vi "Write Tags.vi"(8 "error in (no error)":errorcluster, 11 "State in":T1={"State"=enum."Idle", "Start Time"=timestamp(0 s since 1904-01-01), "Configuration"={"Cycle Period"=0.0, "Mettler"={"VISA resource name"="", "Simulated?"=FALSE}, "Scale Type"=""}, "Current Time"=timestamp(0 s since 1904-01-01), "First Iteration"=FALSE, "Data"={"Scale Read(g)"=0.0}, "Process Name"="", "Log Started"=FALSE}) -> (0 "error out":errorcluster, 3 "State out":T1={"State"=enum."Idle", "Start Time"=timestamp(0 s since 1904-01-01), "Configuration"={"Cycle Period"=0.0, "Mettler"={"VISA resource name"="", "Simulated?"=FALSE}, "Scale Type"=""}, "Current Time"=timestamp(0 s since 1904-01-01), "First Iteration"=FALSE, "Data"={"Scale Read(g)"=0.0}, "Process Name"="", "Log Started"=FALSE})   [LabVIEW 2018, in "Scale Module.lvlib" / "Scale Module Engine.lvlib"]
uses:
  Scale Module Engine.lvlib
  State Cluster.ctl
  State Enum.ctl
  Feed Module/Controls/Scale Module Settings Cluster.ctl
  Mettler Toledo/Controls/Settings Cluster.ctl
  Tag VIs/Tag FGV Operation Enum.ctl
  Shared Variables/Dynamic Shared Variables.lvlib
  Scale Module.lvlib
  Mettler Toledo/Mettler Toledo.lvlib
panel:
  # "Scale Settings"
  # "Scale Settings"
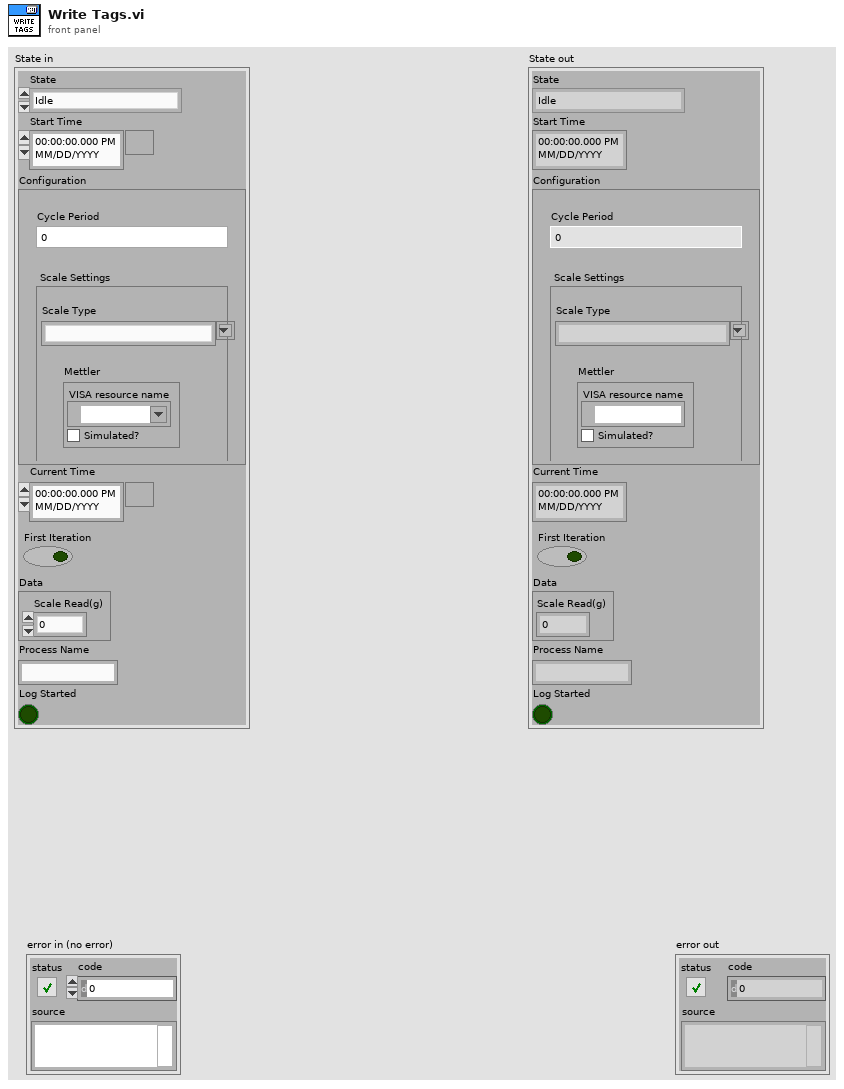
[diagram p1: front panel]
types:
  T1 = typedef "Scale Module.lvlib/Scale Module Engine.lvlib/State Cluster.ctl" = cluster{"State":T2, "Start Time":timestamp, "Configuration":T3, "Current Time":timestamp, "First Iteration":bool, "Data":cluster{"Scale Read(g)":dbl}, "Process Name":string, "Log Started":bool}
  T2 = typedef "Scale Module.lvlib/Scale Module Engine.lvlib/State Enum.ctl" = enum16{"Measuring", "Idle"}
  T3 = typedef "Scale Module.lvlib/Scale Module Settings Cluster.ctl" = cluster{"Cycle Period":dbl, "Mettler":T4, "Scale Type":string}
  T4 = typedef "Mettler Toledo.lvlib/Settings Cluster.ctl" = cluster{"VISA resource name":refnum<visa-resource-name>, "Simulated?":bool}
  T5 = typedef "Tag FGV Operation Enum.ctl" = enum16{"Init", "Set Notification Queue", "Create Tag", "Commit", "Write Tag (Numeric)", "Write Tag (Boolean)", "Read All Tags", "Read One Tag", "Delete Tag Category", "Set Alarm Parameters (Numeric)", "Set Alarm Parameters (Boolean)", "Enable All Alarms", "Disable All Alarms", "Delete All Tags", "Read Alarms", "Ack Alarm", "Read Alarm Parameters (Numeric)", "Read Alarm Parameters (Boolean)"}
  T6 = cluster{"Scale Tag":string, "Output Device Tag":string}
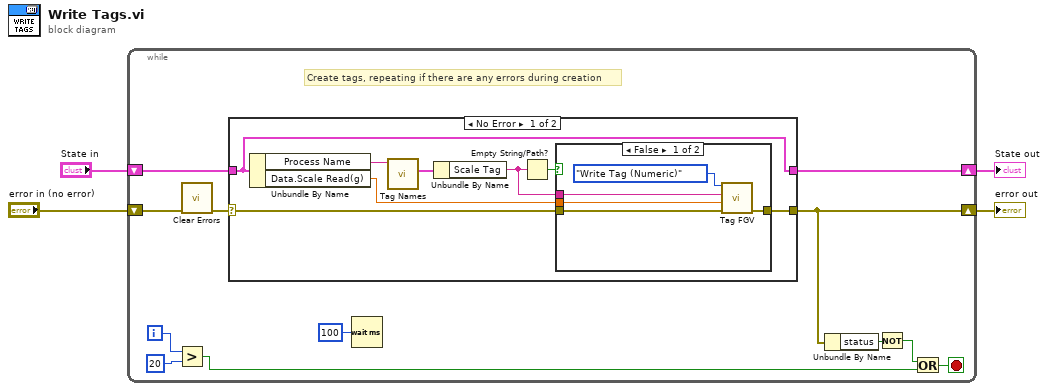
[diagram p0: block diagram]
diagram:
  n1 = while {
    shift-right: [w9] -> w3
    shift-left: "error in (no error)" -> [w14]
    shift-right: [w15] -> w1
    shift-left: "State in" -> [w16]
    i -> [w7]
    stop <- w10 stop-if-true
    # "Create tags, repeating if there are any errors during creation"
    n2 = Greater?(x=w7, y=20) -> (0:w5:bool)
    n3 = call <vilib>:"Clear Errors.vi"("error in (no error)"=w14) -> ("error out"=w13:errorcluster)  [unwired: 5 in, 1 out]
    n4 = case shown="No Error" w13 {
      selector: w13 -> [w21 w32]
      tunnel: [w24 w32] -> w9
      tunnel: w16 -> [w22 w31]
      tunnel: [w22 w31] -> w15
      frame No Error {
        n5 = Unbundle By Name(w22) -> ("Process Name"=w17:string, "Data.Scale Read(g)"=w20:dbl)
        n6 = call "Tag Names.vi"("Process Name"=w17) -> ("Scale Tags"=w19:T6)  [unwired: 8 in, 2 out]
        n7 = Unbundle By Name(w19) -> ("Scale Tag"=w18:string)
        n8 = Empty String/Path?(string/path=w18) -> (empty?=w23:bool)
        n9 = case shown="False" w23 {
          tunnel: [w29 w30] -> w24
          tunnel: w21 -> [w28 w30]
          tunnel: w20 -> [w25 _]
          tunnel: w18 -> [w26 _]
          frame False {
            n10 = call "Tag FGV.vi"("Operation"=Tag_FGV_Operation_Enum."Write Tag (Numeric)", "Tag Name"=w26, "Data"=w25, "error in (no error)"=w28) -> ("error out"=w29:errorcluster)  [unwired: 4 in, 7 out]
          }
          frame True {
          }
        }
      }
      frame Error {
      }
    }
    n11 = Wait (ms)(milliseconds to wait=u32 100) -> ()  [unwired: 1 out]
    n12 = Unbundle By Name(w9) -> ("status"=w11:bool)
    n13 = Not(x=w11) -> (.not. x?=w12:bool)
    n14 = Or(x=w12, y=w5) -> (x .or. y?=w10:bool)
  }
  "error out" <- w3
  "State out" <- w1
